vi "testIterationCountMismatch.vi"(8 "error in (no error)":errorcluster, 11 "TestCase in":refnum<class "TestPBKDF2.lvclass">) -> (0 "error out":errorcluster, 3 "TestCase out":refnum<class "TestPBKDF2.lvclass">)   [LabVIEW 2021, in "TestPBKDF2.lvclass"]
uses:
  TestPBKDF2.lvclass
  Asymmetric Encryption/RSA/HashingAlgorithm.ctl
  <vilib>/addons/_JKI Toolkits/VI Tester/TestCase.llb/TestCase.lvclass
  Key Derivation/dotNET Crypto Key Derivation.lvlib
  Utility/dotNET Crypto Utility.lvlib
  C:/Program Files (x86)/National Instruments/LabVIEW 2021/vi.lib/addons/_JKI Toolkits/VI Tester/TestCase.llb/TestCase.lvclass
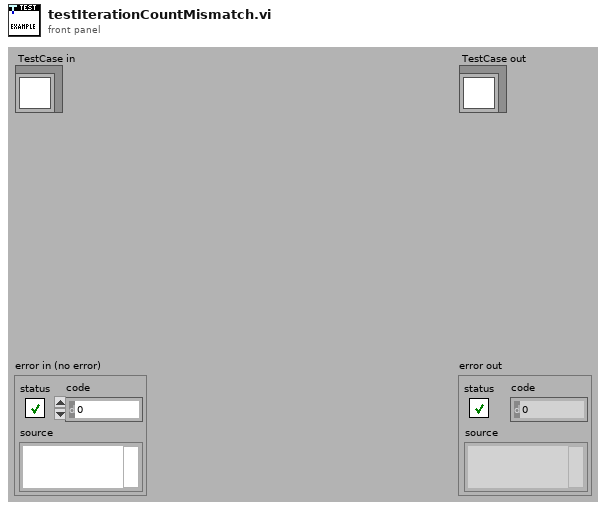
[diagram p1: front panel]
types:
  T1 = typedef "dotNET Crypto Utility.lvlib/HashingAlgorithm.ctl" = enum16{"MD5", "SHA1", "SHA256", "SHA384", "SHA512"}
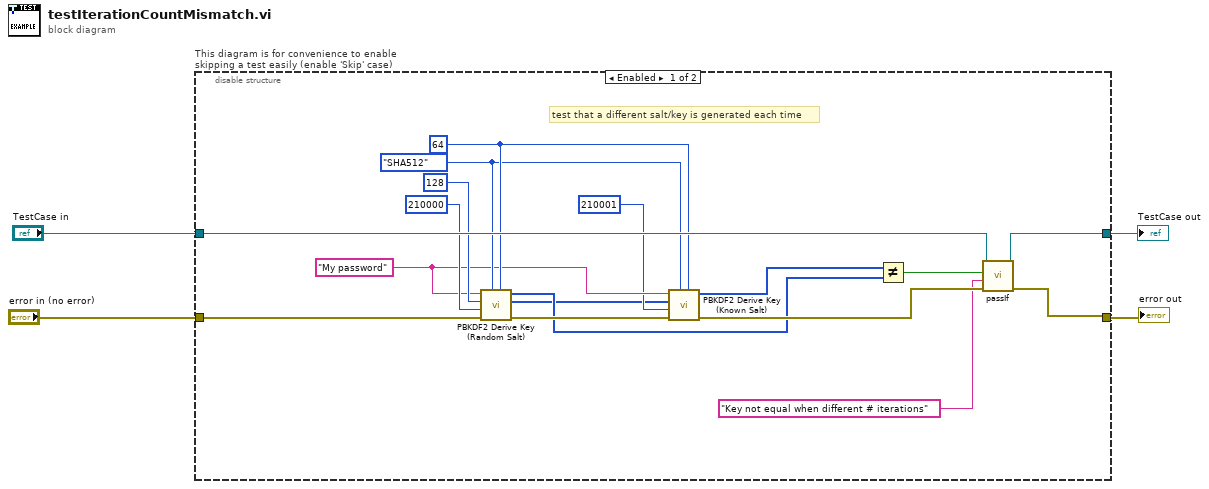
[diagram p0: block diagram]
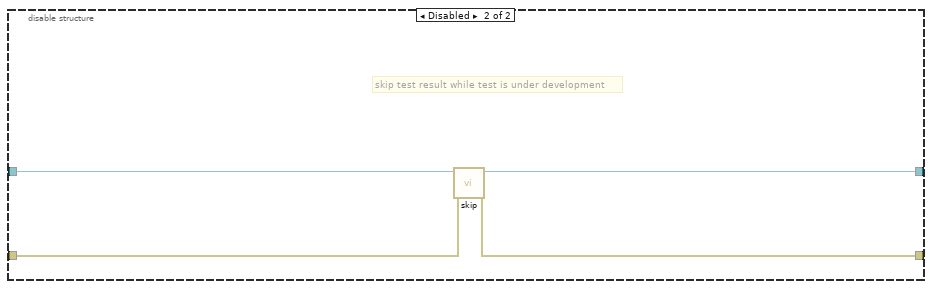
[diagram p2: hidden frame]
diagram:
  n1 = disable-structure "This diagram is for convenience to enable skipping a test easily (enable 'Skip' case)" shown="Enabled" {
    disable-tunnel: "TestCase in" -> [w21 w25]
    disable-tunnel: [w20 w23] -> w1
    disable-tunnel: [w19 w24] -> w3
    disable-tunnel: "error in (no error)" -> [w18 w22]
    frame Enabled {
      w11 = "My password" ("Password")
      w14 = HashingAlgorithm."SHA512" ("HashingAlgorithm (SHA512)")
      w15 = 64 ("Key length (64 bytes)")
      # "test that a different salt/key is generated each time"
      n2 = call "PBKDF2 Derive Key (Random Salt).vi"("Key length (64 bytes)"=w15, "HashingAlgorithm (SHA512)"=w14, "error in (no error)"=w18, "iterations (210000)"=210000, "saltSize (128)"=128, "Password"=w11) -> ("error out"=w17:errorcluster, "Salt"=w6:u8[], "Derived Key"=w9:u8[])  [unwired: 3 in]
      n3 = call "PBKDF2 Derive Key (Known Salt).vi"("Key length (64 bytes)"=w15, "HashingAlgorithm (SHA512)"=w14, "error in (no error)"=w17, "iterations (210000)"=210001, "Salt"=w6, "Password"=w11) -> ("error out"=w16:errorcluster, "Derived Key"=w10:u8[])  [unwired: 4 in]
      n4 = Not Equal?(x=w10, y=w9) -> (x != y?=w5:bool)
      n5 = call-dynamic "passIf.vi"("error in (no error)"=w16, "message (\"\")"="Key not equal when different # iterations" ("message (\"\")"), "pass"=w5, "TestCase in"=w21) -> ("error out"=w19:errorcluster, "TestCase out"=w20:refnum<class "TestPBKDF2.lvclass">)  [unwired: 6 in]
    }
    frame Disabled {
      # "skip test result while test is under development"
      n6 = call <vilib>:"skip.vi"("error in (no error)"=w22, "TestCase in"=w25) -> ("error out"=w24:errorcluster, "TestCase out"=w23:refnum<class "TestPBKDF2.lvclass">)  [unwired: 8 in]
    }
  }
  "error out" <- w3
  "TestCase out" <- w1
